vi "Parse Config File.vi"(8 "error in (no error)":errorcluster, 11 "Filtered Config Entries":string="1737340154015584000\ttest\tCreate\tTemplatePlugin.0.2.3.lvlibp:TemplatePlugin.lvclass\t<version> 0.2.3.0\t\n1737340198541890000\ttest\tConfigure\t{\"Common\":{\"Period (s)\":0.001,\"Offset (us)\":0,\"ClockID\":0,\"Priority\":101,\"Processor\":-2},\"Step\":100}\n1737340326509796000\tlovingit6\tCreate\tCIFCorePlugin.0.1.2.lvlibp:CIFCorePlugin.lvclass\t<version> 0.1.2.0\t\n1737340326559504000\tchannelme\tCreate\tTemplatePlugin.0.2.3.lvlibp:TemplatePlugin.lvclass\t<version> 0.2.3.0\t\n1737340326827852000\tchannelme\tConnect\t<publisher> channelme/doubleout <subscriber> channelme/doublein1 <data> \n1737340326835711000\tchannelme\tConfigure\t{\"Common\":{\"Period (s)\":0.001,\"Offset (us)\":0,\"ClockID\":0,\"Priority\":101,\"Processor\":-2},\"Step\":100}\n1737340327017380000\tlovingit6\tRun\n") -> (0 "error out":errorcluster, 2 "Logic Entries":string[](array[string]), 3 "Configuration Entries":string[](array[string]))   [LabVIEW 2021, in "Python Orchestration.lvlib"]
uses:
  Python Orchestration.lvlib
  CIFCore/Common/Typedef/Errors.ctl
  Typedef/Scripted Line.ctl
  <vilib>/CIF Foundation/CIF Utilities/Errors/Append Error Location.vi
  <vilib>/string/Create NI GUID.vi
  CIFCore/Common/CIFCoreCommon.lvlib
panel:
  out "Array 5":string[](array[string])
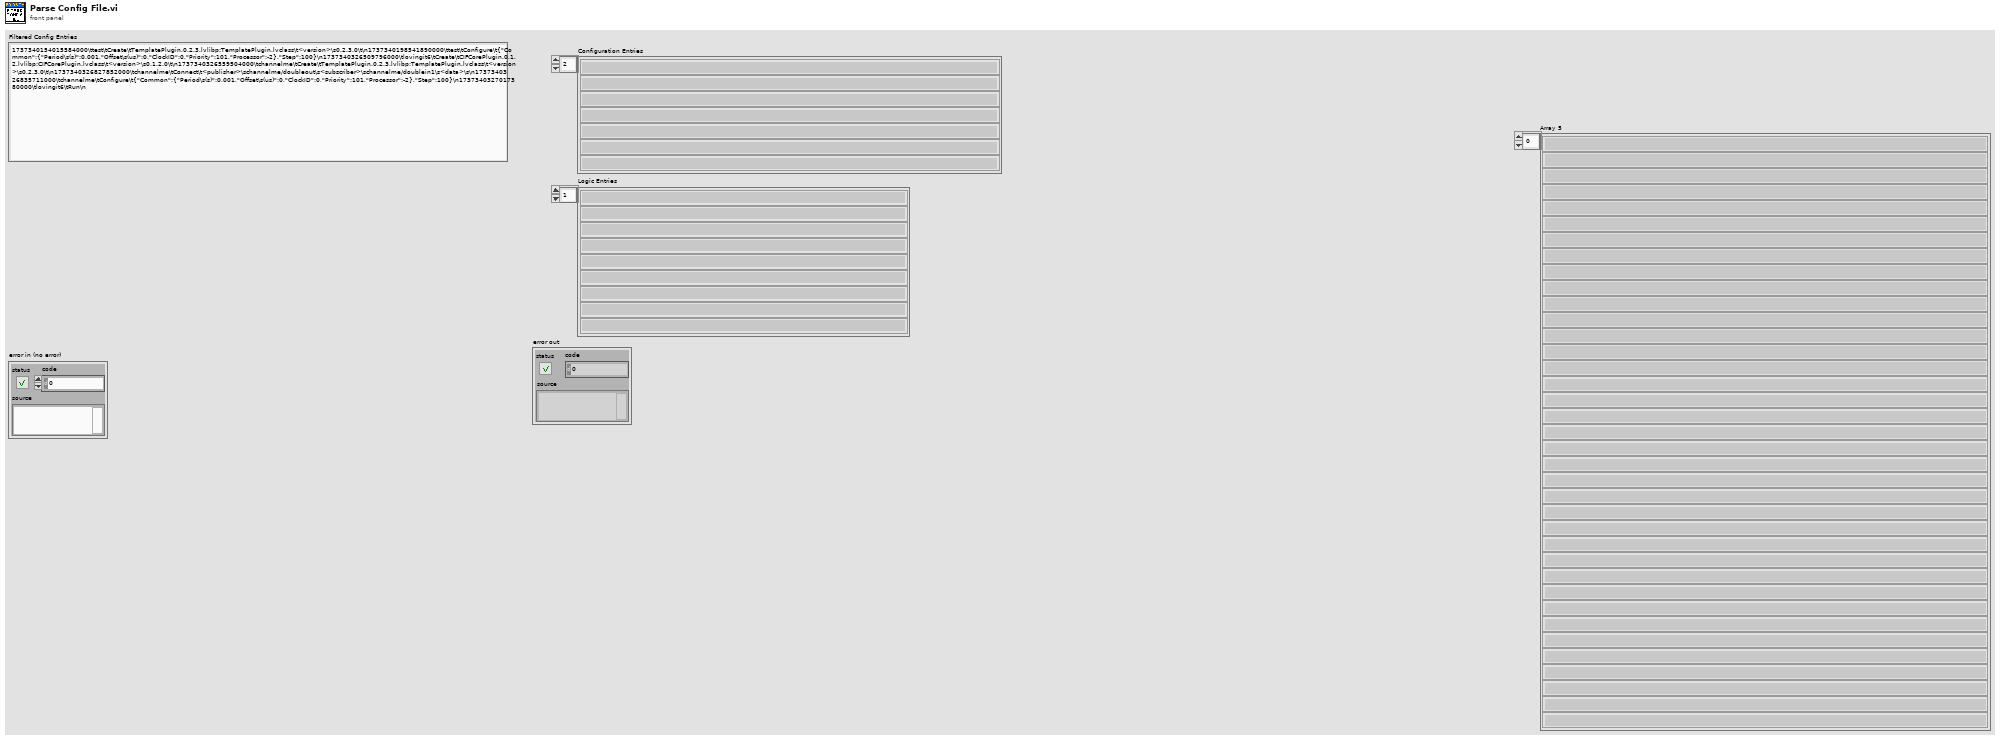
[diagram p1: front panel]
types:
  T1 = typedef "CIFCoreCommon.lvlib/Errors.ctl" = enum16{"Invalid Clock ID", "Long Sleep", "gRPC Server Not Found", "Config Parse", "Timestamp Wrap", "Delayed Execution", "Duplicate Channel", "Missing Channel", "Incorrect Type", "Flatten Error", "Unflatten Data", "Unique Name", "Plugin Not Found", "Plugin Type Not Found", "Plugin Version Not Found", "Manager Not Found", "Numerical Issue", "Time Jump", "Clock ID Match", "Channel Length", "Plugin Connection", "gRPC Server Connection", "PPL Name Match", "Build", "Config Log Parse", "Plugin Load", "UI Subpanel Load", "Python Name", "Invalid Name"}
  T2 = typedef "Python Orchestration.lvlib/Scripted Line.ctl" = cluster{"Entry":string, "Valid":bool}
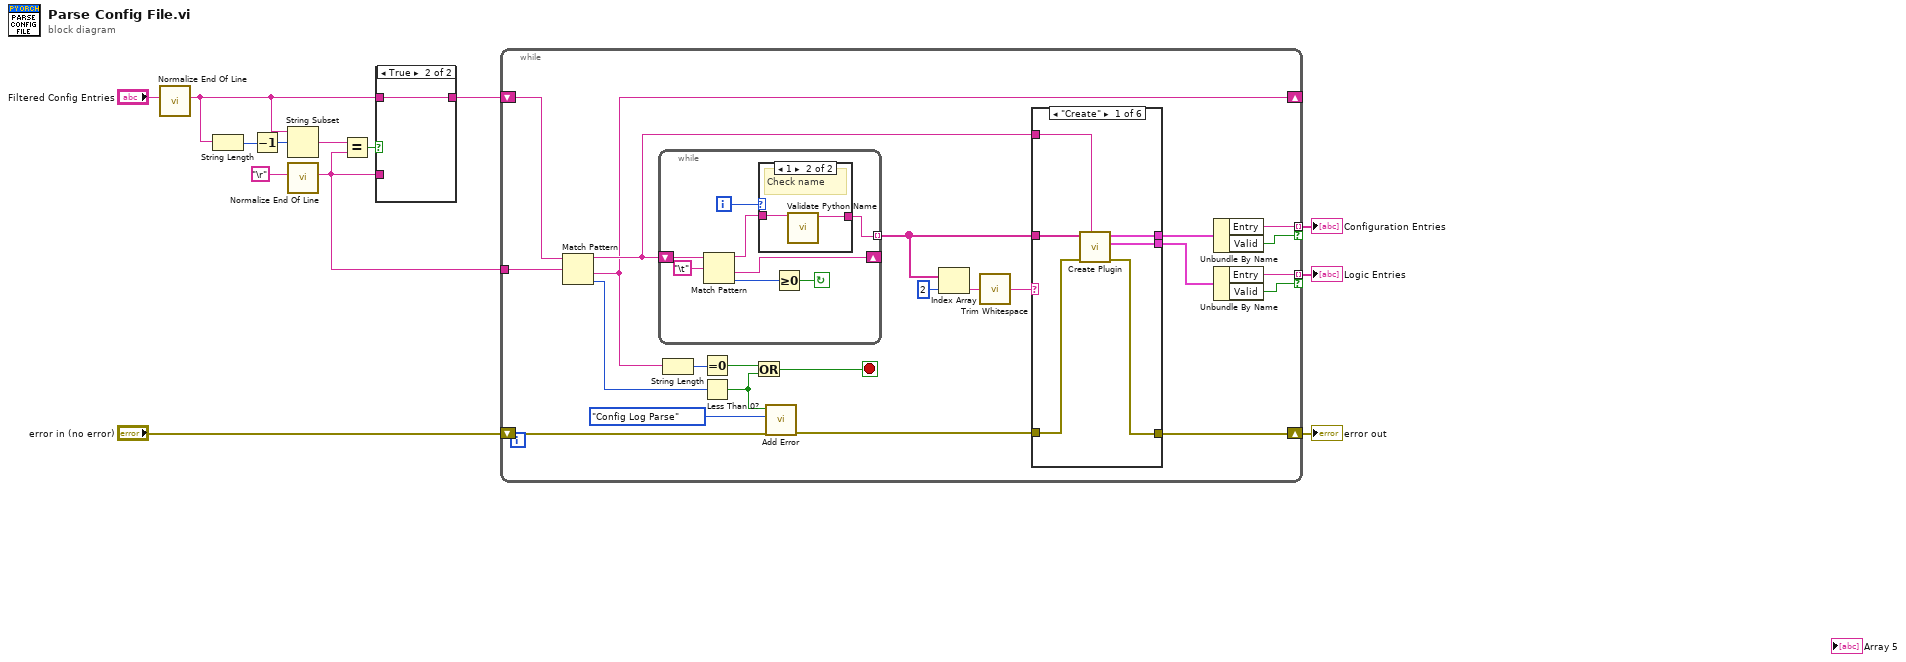
[diagram p0: block diagram]
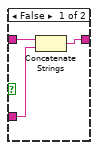
[diagram p2: hidden frame]
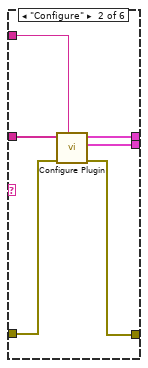
[diagram p3: hidden frame]
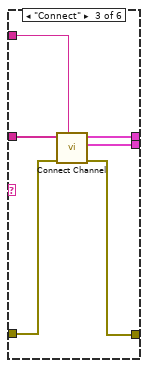
[diagram p4: hidden frame]
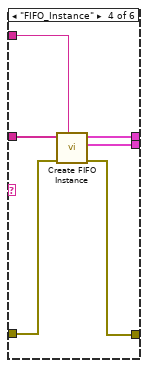
[diagram p5: hidden frame]
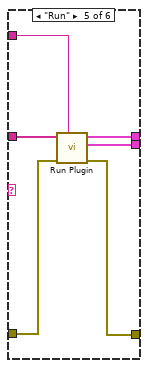
[diagram p6: hidden frame]
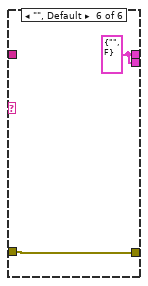
[diagram p7: hidden frame]
diagram:
  n1 = call <vilib>:"Normalize End Of Line.vi"("string in"="Filtered Config Entries") -> ("string out"=w3:string)  [unwired: 7 in]
  n2 = String Length(string=w3) -> (length=w9:i32)
  n3 = Decrement(x=w9) -> (x-1=w8:i32)
  n4 = String Subset(string=w3, offset (0)=w8) -> (substring=w5:string)  [unwired: 1 in]
  n5 = call <vilib>:"Normalize End Of Line.vi"("string in"="\r") -> ("string out"=w1:string)  [unwired: 7 in]
  n6 = Equal?(x=w5, y=w1) -> (x = y?=w4:bool)
  n7 = case shown="True" w4 {
    tunnel: w1 -> [w16 _]
    tunnel: w3 -> [w15 w17]
    tunnel: [w14 w17] -> w2
    frame False {
      n8 = Concatenate Strings(w15, w16) -> (w14:string)
    }
    frame True {
    }
  }
  n9 = while {
    shift-right: [w23] -> _
    shift-left: w2 -> [w40]
    shift-right: [w29] -> w10
    shift-left: "error in (no error)" -> [w30]
    tunnel: [w19] -> w12 mode=indexing if=w25
    tunnel: [w26] -> w11 mode=indexing if=w24
    tunnel: w1 -> [w18]
    stop <- w31 stop-if-true
    n10 = Match Pattern(string=w40, regular expression=w18) -> (before substring=w38:string, after substring=w23:string, offset past match=w36:i32)  [unwired: 1 in, 1 out]
    n11 = while {
      shift-right: [w78] -> _
      shift-left: w38 -> [w80]
      tunnel: [w73] -> w22 mode=indexing
      i -> [w75]
      stop <- w76 continue-if-true
      n12 = Match Pattern(string=w80, regular expression="\t") -> (before substring=w74:string, after substring=w78:string, offset past match=w77:i32)  [unwired: 1 in, 1 out]
      n13 = case shown="1" w75 {
        tunnel: w74 -> [w81 w83]
        tunnel: [w81 w82] -> w73
        frame 0, Default {
        }
        frame 1 {
          # "Check name"
          n14 = call "Validate Python Name.vi"("Name In"=w83) -> ("Valid Name"=w82:string)  [unwired: 9 in, 1 out]
        }
      }
      n15 = Greater Or Equal To 0?(x=w77) -> (x >= 0?=w76:bool)
    }
    n16 = String Length(string=w23) -> (length=w37:i32)
    n17 = Equal To 0?(x=w37) -> (x = 0?=w35:bool)
    n18 = Less Than 0?(x=w36) -> (x < 0?=w33:bool)
    n19 = Or(x=w35, y=w33) -> (x .or. y?=w31:bool)
    n20 = call "Add Error.vi"("error in (no error)"=w30, "Error"=Errors."Config Log Parse", "Insert Error"=w33) -> ("error out"=w32:errorcluster)  [unwired: 8 in]
    n21 = Index Array(array=w22, index=2) -> (element=w21:string)
    n22 = call <vilib>:"Trim Whitespace.vi"("string"=w21) -> ("trimmed string"=w20:string)  [unwired: 1 in]
    n23 = case shown="\"Create\"" w20 {
      tunnel: w22 -> [w46 w52 w58 w64 w70 _]
      tunnel: w38 -> [w45 w51 w57 w63 w69 _]
      tunnel: w32 -> [w44 w50 w56 w62 w68 w71]
      tunnel: [w43 w49 w55 w61 w67 w71] -> w29
      tunnel: [w42 w48 w54 w59 w66 w72] -> w27
      tunnel: [w41 w47 w53 w60 w65 w72] -> w28
      frame "Create" {
        n24 = call "Create Plugin.vi"("Configuration Entry"=w45, "error in (no error)"=w44, "Configuration Parameters"=w46) -> ("error out"=w43:errorcluster, "Logic Entry"=w41:T2, "Configuration Entry"=w42:T2)  [unwired: 6 in]
      }
      frame "Configure" {
        n25 = call "Configure Plugin.vi"("Configuration Entry"=w51, "error in (no error)"=w50, "Configuration Parameters"=w52) -> ("error out"=w49:errorcluster, "Logic Entry"=w47:T2, "Configuration Entry"=w48:T2)  [unwired: 6 in]
      }
      frame "Connect" {
        n26 = call "Connect Channel.vi"("Configuration Entry"=w57, "error in (no error)"=w56, "Configuration Parameters"=w58) -> ("error out"=w55:errorcluster, "Logic Entry"=w53:T2, "Configuration Entry"=w54:T2)  [unwired: 6 in]
      }
      frame "FIFO_Instance" {
        n27 = call "Create FIFO Instance.vi"("Configuration Entry"=w63, "error in (no error)"=w62, "Configuration Parameters"=w64) -> ("error out"=w61:errorcluster, "Logic Entry"=w60:T2, "Configuration Entry"=w59:T2)  [unwired: 6 in]
      }
      frame "Run" {
        n28 = call "Run Plugin.vi"("Configuration Entry"=w69, "error in (no error)"=w68, "Configuration Parameters"=w70) -> ("error out"=w67:errorcluster, "Logic Entry"=w65:T2, "Configuration Entry"=w66:T2)  [unwired: 6 in]
      }
      frame "", Default {
        w72 = T2 {"Entry"="", "Valid"=FALSE} ("Configuration Entry")
      }
    }
    n29 = Unbundle By Name(w27) -> ("Entry"=w19:string, "Valid"=w25:bool)
    n30 = Unbundle By Name(w28) -> ("Entry"=w26:string, "Valid"=w24:bool)
  }
  "Configuration Entries" <- w12
  "Logic Entries" <- w11
  "error out" <- w10
